vi "基于延迟的串口通信流程.vi"() -> ()   [LabVIEW 2013]
uses:
  <vilib>/Instr/_visa.llb/VISA Configure Serial Port (Instr).vi
panel:
  out "返回数":u32
  out "读取缓冲区":string
  in  "查询":string(combo)="CH0"
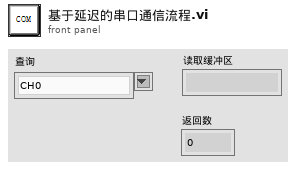
[diagram p1: front panel]
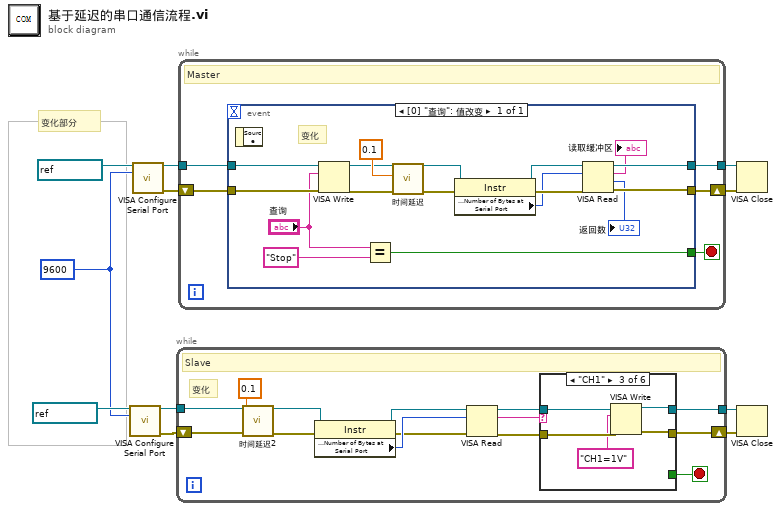
[diagram p0: block diagram]
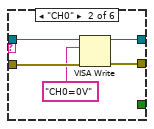
[diagram p3: hidden frame]
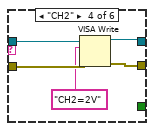
[diagram p4: hidden frame]
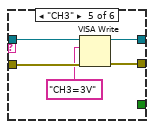
[diagram p5: hidden frame]
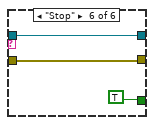
[diagram p6: hidden frame]
diagram:
  w5 = u32 9600 ("baud rate (9600)")
  # "变化部分"
  n1 = call-poly "VISA Configure Serial Port"("VISA resource name"=refnum<visa-resource-name> "COM3", "baud rate (9600)"=w5) -> ("VISA resource name out"=w3:refnum<visa-resource-name>, "error out"=w4:errorcluster)  [unwired: 12 in]
  n2 = call-poly "VISA Configure Serial Port"("VISA resource name"=refnum<visa-resource-name> "COM2", "baud rate (9600)"=w5) -> ("VISA resource name out"=w10:refnum<visa-resource-name>, "error out"=w9:errorcluster)  [unwired: 12 in]
  n3 = while "While循环" {
    tunnel: w3 -> [w22]
    shift-right: [w13] -> w1
    shift-left: w4 -> [w24]
    tunnel: [w15] -> w2
    stop <- w12 stop-if-true
    # "变化"
    # "Slave"
    n4 = call "时间延迟2"("error in (no error)"=w24, "Delay Time (s)"=0.1) -> ("error out"=w21:errorcluster)  [unwired: 9 in]
    n5 = property class="Instr"(reference=w22, error in=w21) -> (reference out=w20:refnum<visa-resource-name>, error out=w18:errorcluster, "Serial Settings:Number of Bytes at Serial Port"=w19:u32)
    n6 = VISA Read(VISA resource name=w20, byte count=w19, error in (no error)=w18) -> (VISA resource name out=w16:refnum<visa-resource-name>, read buffer=w17:string, error out=w14:errorcluster)  [unwired: 1 out]
    n7 = case shown="\"CH1\"" w17 {
      tunnel: w16 -> [w26 w30 w35 w40 w45 w49]
      tunnel: [w26 w28 w33 w38 w43 w49] -> w15
      tunnel: w14 -> [w25 w31 w36 w41 w46 w48]
      tunnel: [w25 w27 w32 w37 w42 w48] -> w13
      tunnel: [_ _ _ _ _ TRUE] -> w12
      frame "", Default {
      }
      frame "CH0" {
        n8 = VISA Write(VISA resource name=w30, write buffer="CH0=0V" ("写入缓冲区"), error in (no error)=w31) -> (VISA resource name out=w28:refnum<visa-resource-name>, error out=w27:errorcluster)  [unwired: 1 out]
      }
      frame "CH1" {
        n9 = VISA Write(VISA resource name=w35, write buffer="CH1=1V" ("写入缓冲区"), error in (no error)=w36) -> (VISA resource name out=w33:refnum<visa-resource-name>, error out=w32:errorcluster)  [unwired: 1 out]
      }
      frame "CH2" {
        n10 = VISA Write(VISA resource name=w40, write buffer="CH2=2V" ("写入缓冲区"), error in (no error)=w41) -> (VISA resource name out=w38:refnum<visa-resource-name>, error out=w37:errorcluster)  [unwired: 1 out]
      }
      frame "CH3" {
        n11 = VISA Write(VISA resource name=w45, write buffer="CH3=3V" ("写入缓冲区"), error in (no error)=w46) -> (VISA resource name out=w43:refnum<visa-resource-name>, error out=w42:errorcluster)  [unwired: 1 out]
      }
      frame "Stop" {
      }
    }
  }
  n12 = while {
    tunnel: w10 -> [w51]
    shift-right: [w52] -> w8
    shift-left: w9 -> [w53]
    tunnel: [w50] -> w7
    stop <- w54 stop-if-true
    # "Master"
    n13 = event shown="[0] \"查询\": 值改变" {
      selector: _ -> [_]
      dyn-events: _ -> [_]
      timeout: _ -> [_]
      tunnel: [w55] -> w54
      tunnel: w53 -> [w70]
      tunnel: [w60] -> w52
      tunnel: w51 -> [w69]
      tunnel: [w63] -> w50
      event "查询": Value Change {
        # "变化"
        n14 = event-data() -> ()  [unwired: 1 in, 1 out]
        n15 = VISA Write(VISA resource name=w69, write buffer="查询", error in (no error)=w70) -> (VISA resource name out=w65:refnum<visa-resource-name>, error out=w67:errorcluster)  [unwired: 1 out]
        n16 = Equal?(x="查询", y="Stop") -> (x = y?=w55:bool)
        n17 = call "时间延迟"("error in (no error)"=w67, "Delay Time (s)"=0.1) -> ("error out"=w66:errorcluster)  [unwired: 9 in]
        n18 = property class="Instr"(reference=w65, error in=w66) -> (reference out=w64:refnum<visa-resource-name>, error out=w62:errorcluster, "Serial Settings:Number of Bytes at Serial Port"=w61:u32)
        n19 = VISA Read(VISA resource name=w64, byte count=w61, error in (no error)=w62) -> (VISA resource name out=w63:refnum<visa-resource-name>, read buffer=→"读取缓冲区":string, return count=→"返回数":u32, error out=w60:errorcluster)
      }
    }
  }
  n20 = VISA Close(VISA resource name=w7, error in (no error)=w8) -> ()  [unwired: 1 out]
  n21 = VISA Close(VISA resource name=w2, error in (no error)=w1) -> ()  [unwired: 1 out]
